vi "Get Fast Tree Level Keys.vi"(9 "error in (no error)":errorcluster) -> (1 "error out":errorcluster, 2 "Level Down Keys":string[](array[string])=["ENDEL", "ENDSTR"], 3 "Level Up Keys":string[](array[string])=["BGNSTR", "AREF", "BOUNDARY", "BOX", "NODE", "PATH", "SREF", "TEXT"])   [LabVIEW 2019, in "ParseGDSII.lvclass"]
uses:
  ParseGDSII.lvclass
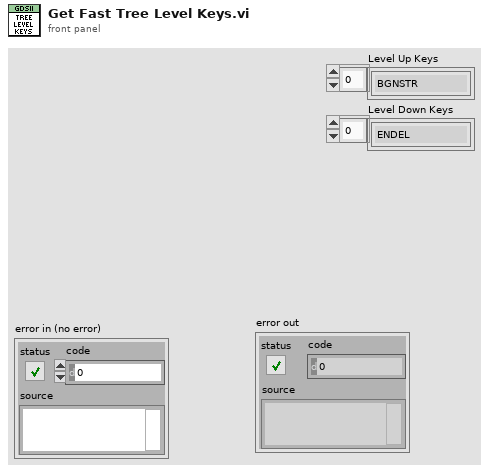
[diagram p1: front panel]
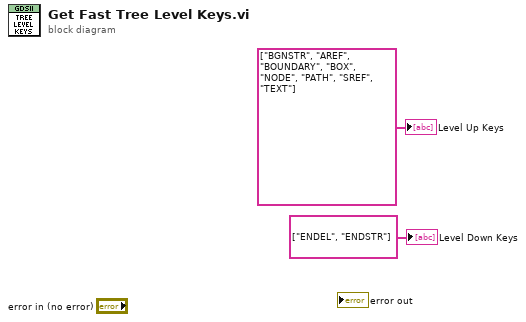
[diagram p0: block diagram]
diagram:
  "Level Up Keys" <- string[] ["BGNSTR", "AREF", "BOUNDARY", "BOX", "NODE", "PATH", "SREF", "TEXT"]
  "Level Down Keys" <- string[] ["ENDEL", "ENDSTR"]
